vi "Actor Core.vi"(8 "error in":errorcluster, 11 "VG-VNA_GUI in":refnum<class "VG-VNA_GUI.lvclass">) -> (0 "error out":errorcluster, 3 "Actor out":refnum<class "Actor.lvclass">)   [LabVIEW 2020, in "VG-VNA_GUI.lvlib" / "VG-VNA_GUI.lvclass"]
doc: "(<B>Filename</B>: Actor Framework.lvlib:Actor.lvclass:Actor Core.vi)\n\nReceives messages to the actor, reacts to them, and initiates any error handling that may shut the actor down.\n\nDescendant classes may override this VI to append parallel tasks for the actor to complete while it handles messages. Overrides use the Call Parent Class Method node."
uses:
  VG-VNA_GUI.lvclass
  C:/Program Files (x86)/National Instruments/LabVIEW 2020/vi.lib/ActorFramework/Actor/Actor.lvclass
  <vilib>/ActorFramework/Actor/Actor.lvclass
  classes/vna-drivers/liteVNA/VD-connection_settings.ctl
  classes/hardware-protocol/serial/HP-S-baudrate.ctl
  classes/vna-drivers/liteVNA/VD-settingsEasy.ctl
  classes/vna-drivers/liteVNA/VD-sampleSize.ctl
  VG-main_tab.ctl
  VG-sec_tab.ctl
  classes/vna-drivers/liteVNA/VD-settings_status.ctl
  data_handler/VDH-VNA_data_handler/VDH-VNA_data_handler/VDH-calibration_status.ctl
  data_handler/VDH-VNA_data_handler/VDH-VNA_data_handler/VDH-SOLT_calib_Status.ctl
  data_handler/VDH-VNA_data_handler/VDH-VNA_data_handler/VDH-Calibration_prosess.ctl
  data_handler/VDH-VNA_data_handler/VDH-VNA_data_handler/VDH-Calibration_enum.ctl
  hardware_manager/VHM-VNA_Hardware_Manager/VHM-VNA_Hardware_Manager/VHM-connection_status.ctl
  hardware_manager/VHM-VNA_Hardware_Manager/VHM-VNA_Hardware_Manager/VHM-continuous_get_clust.ctl
  VG-file_name_choices.ctl
  VG-data_format_selector.ctl
  VG-VNA_GUI.lvclass/VG-VNA_GUI.ctl
  hardware_manager/VHM-VNA_Hardware_Manager/VHM-VNA_Hardware_Manager Messages/VHM-connectionSettings Msg/VHM-connectionSettings Msg.lvclass/VHM-connectionSettings Msg.ctl
  <vilib>/ActorFramework/Message Enqueuer/Message Enqueuer.lvclass/Message Enqueuer.ctl
  hardware_manager/VHM-VNA_Hardware_Manager/VHM-VNA_Hardware_Manager Messages/VHM-continiousDataSet Msg/VHM-continiousDataSet Msg.lvclass/VHM-continiousDataSet Msg.ctl
  hardware_manager/VHM-VNA_Hardware_Manager/VHM-VNA_Hardware_Manager Messages/VHM-setSettings Msg/VHM-setSettings Msg.lvclass/VHM-setSettings Msg.ctl
  data_handler/VDH-VNA_data_handler/VDH-VNA_data_handler Messages/VDH-loadCalibration Msg/VDH-loadCalibration Msg.lvclass/VDH-loadCalibration Msg.ctl
  data_handler/VDH-VNA_data_handler/VDH-VNA_data_handler/VDH-save_parameters.ctl
  data_handler/VDH-VNA_data_handler/VDH-VNA_data_handler Messages/VDH-RequestSaveData Msg/VDH-RequestSaveData Msg.lvclass/VDH-RequestSaveData Msg.ctl
  data_handler/VDH-VNA_data_handler/VDH-VNA_data_handler Messages/VDH-storeCalibration Msg/VDH-storeCalibration Msg.lvclass/VDH-storeCalibration Msg.ctl
  <vilib>/ActorFramework/Actor/Actor.lvclass/Actor.ctl
  <vilib>/ActorFramework/Message Enqueuer/Enqueue.vi
  <vilib>/ActorFramework/Message Enqueuer/Init from Existing Queue.vi
  hardware_manager/VHM-VNA_Hardware_Manager/VHM-VNA_Hardware_Manager Messages/VHM-connectionSettings Msg/VHM-connectionSettings Msg.lvclass
  C:/Program Files (x86)/National Instruments/LabVIEW 2020/vi.lib/ActorFramework/Message/Message.lvclass
  hardware_manager/VHM-VNA_Hardware_Manager/VHM-VNA_Hardware_Manager Messages/VHM-connect Msg/VHM-connect Msg.lvclass
  hardware_manager/VHM-VNA_Hardware_Manager/VHM-VNA_Hardware_Manager Messages/VHM-getDataSet Msg/VHM-getDataSet Msg.lvclass
  hardware_manager/VHM-VNA_Hardware_Manager/VHM-VNA_Hardware_Manager Messages/VHM-continiousDataSet Msg/VHM-continiousDataSet Msg.lvclass
  hardware_manager/VHM-VNA_Hardware_Manager/VHM-VNA_Hardware_Manager Messages/VHM-disconnect Msg/VHM-disconnect Msg.lvclass
  hardware_manager/VHM-VNA_Hardware_Manager/VHM-VNA_Hardware_Manager Messages/VHM-setSettings Msg/VHM-setSettings Msg.lvclass
  data_handler/VDH-VNA_data_handler/VDH-VNA_data_handler Messages/VDH-generateCalibrationSOLT Msg/VDH-generateCalibrationSOLT Msg.lvclass
  data_handler/VDH-VNA_data_handler/VDH-VNA_data_handler Messages/VDH-loadCalibration Msg/VDH-loadCalibration Msg.lvclass
  data_handler/VDH-VNA_data_handler/VDH-VNA_data_handler Messages/VDH-RequestSaveData Msg/VDH-RequestSaveData Msg.lvclass
  data_handler/VDH-VNA_data_handler/VDH-VNA_data_handler Messages/VDH-RequestStopSaveData Msg/VDH-RequestStopSaveData Msg.lvclass
  data_handler/VDH-VNA_data_handler/VDH-VNA_data_handler Messages/VDH-storeCalibration Msg/VDH-storeCalibration Msg.lvclass
  <vilib>/ActorFramework/Stop Msg/Stop Msg.lvclass
  <vilib>/ActorFramework/Message Priority Queue/Priority Enqueue.vi
  <userlib>/_OpenG.lib/file/file.llb/Valid Path - Traditional__ogtk.vi
  <vilib>/ActorFramework/Message Enqueuer/Message Enqueuer.lvclass
  classes/vna-drivers/liteVNA/VD-LV-LiteVNA.lvclass
  data_handler/VDH-VNA_data_handler/VDH-VNA_data_handler/VDH-VNA_data_handler.lvclass
  hardware_manager/VHM-VNA_Hardware_Manager/VHM-VNA_Hardware_Manager/VHM-VNA_Hardware_Manager.lvclass
  common/features/CF-common_features.lvlib
  <userlib>/_OpenG.lib/file/file.llb/openg_file.lvlib
  classes/hardware-protocol/serial/HP-S-Serial.lvclass
panel:
  in  "Tab Control":enum32{"Main", "Graph"}(tab)
  in  "Main Tab":T1
  in  "autosetup":bool
  in  "connection settings":T2={"Com"="", "baud rate (9600)"=38400} {"baud rate (9600)" items=["75"=75, "110"=110, "134"=134, "150"=150, "300"=300, "600"=600, "1200"=1200, "1800"=1800, "2400"=2400, "4800"=4800, "7200"=7200, "9600"=9600, "14400"=14400, "19200"=19200, "28800"=28800, "38400"=38400, "56000"=56000, "57600"=57600, "115200"=115200, "128000"=128000, "230400"=230400]}
  in  "Connect":bool
  in  "Disconnect":bool
  in  "Set connection settings":bool
  out "connection status":T4
  in  "get set":bool
  in  "Size in sets (0=Until stop)":u8=1
  in  "Stop Reading":bool
  in  "Start Reading":bool
  in  "Stop Saving":bool
  in  "Save Data":bool
  out "Saving Data":bool
  in  "settings":T5={"Start [hz]"=1000000, "Stop [hz]"=5000000, "sampleSize"=101} {"sampleSize" items=["101"=101, "201"=201, "401"=401, "601"=601, "801"=801, "1001"=1001]; "Stop [hz]" format="%.0p"; "Start [hz]" format="%.0p"}
  in  "Set Settings":bool
  in  "Saving name":string="noname"
  in  "Saving path":path
  in  "get cont set":bool
  in  "Read Option":T7
  in  "Second Tab":T8
  in  "calib File Path":path
  in  "Load Calibration file":bool
  out "Calibration Status":T9={"Calib Status"={"Short"=FALSE, "Open"=FALSE, "Load"=FALSE, "Through"=FALSE}, "Calibrated?"=FALSE, "Permativity?"=FALSE, "Progress"={"Progress"=FALSE, "current"=enum."Short", "samples to get"=0}}
  in  "T":bool
  in  "L":bool
  in  "O":bool
  in  "S":bool
  in  "Gen Calib":bool
  in  "Refresh Filename":bool
  out "Filepath":path
  in  "file name choises":T13={"Date"=TRUE, "Time"=TRUE, "Measurement settings"=TRUE, "SOLT?"=TRUE}
  out "File name":string="default_calibration_name"
  in  "Custom filename Part":string
  in  "Save Calibration":bool
  in  "comment":string="Comment"
  in  "Calibration folder Path":path
  out "XY Graph":cluster{u64[], dbl[]}[](graph)
  out "XY Graph 2":cluster{u64[], dbl[]}[](graph)
  out "Settings status":T14
  in  "data format":T15
  in  "Tab Control 2":enum32{"Page 1", "Page 2"}(tab)
  out "XY Graph 3":cluster{u64[], dbl[]}[](graph)
  out "Smith Plot":picture
  out "size(s)":i32
  out "Connected?":bool
  in  "Stop":bool
  out "error IO":errorcluster
  out "current time":timestamp
  # "Manual"
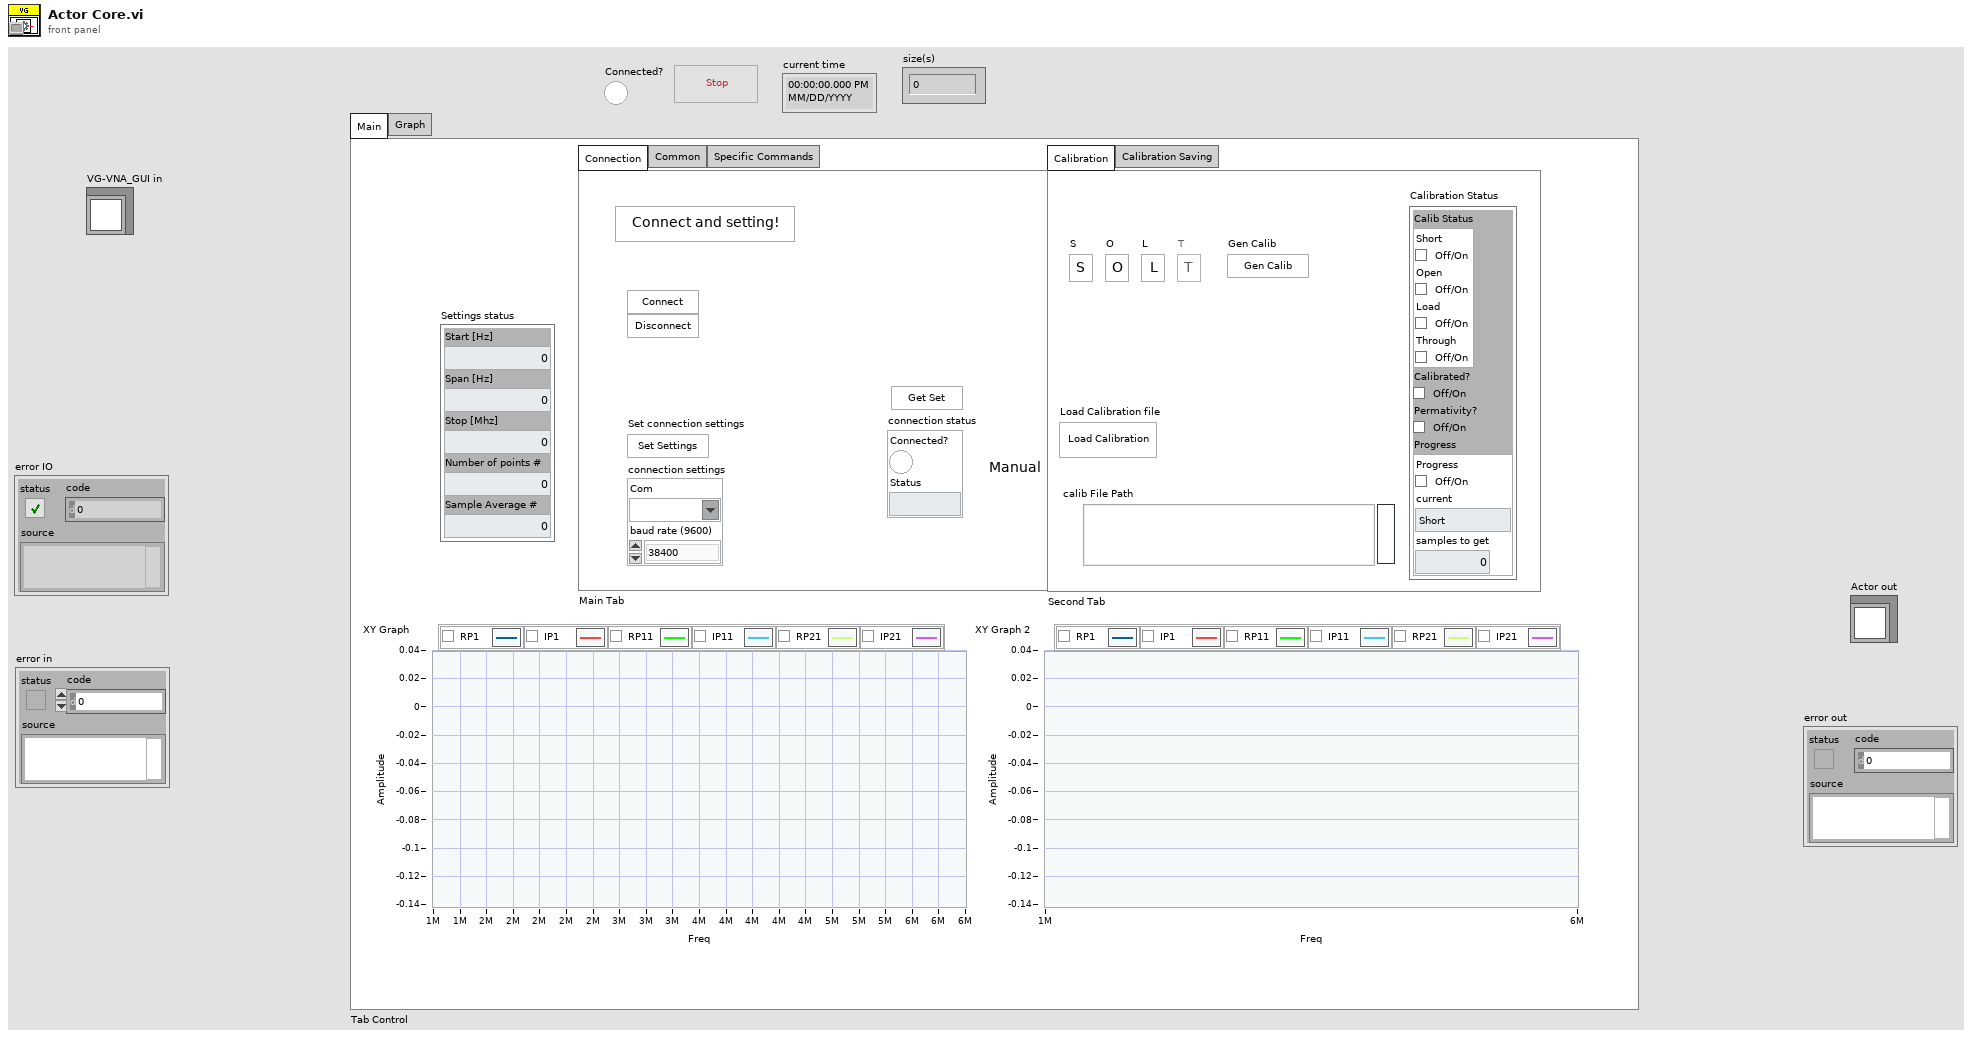
[diagram p1: front panel]
types:
  T1 = typedef "VG-VNA_GUI.lvlib/VG-VNA_GUI.lvclass/VG-main_tab.ctl" = enum32{"Connection", "Common", "Specific Commands"}
  T2 = typedef "VD-LV-LiteVNA.lvclass/VD-connection_settings.ctl" = cluster{"Com":refnum<visa-resource-name>, "baud rate (9600)":T3}
  T3 = typedef "HP-S-Serial.lvclass/HP-S-baudrate.ctl" = u32
  T4 = typedef "VHM-VNA_Hardware_Manager.lvlib/VHM-VNA_Hardware_Manager.lvclass/VHM-connection_status.ctl" = cluster{"Connected?":bool, "Status":string}
  T5 = typedef "VD-LV-LiteVNA.lvclass/VD-settingsEasy.ctl" = cluster{"Start [hz]":u64, "Stop [hz]":u64, "sampleSize":T6}
  T6 = typedef "VD-LV-LiteVNA.lvclass/VD-sampleSize.ctl" = u16
  T7 = typedef "VHM-VNA_Hardware_Manager.lvlib/VHM-VNA_Hardware_Manager.lvclass/VHM-continuous_get_clust.ctl" = cluster{"Amount(0=Continious)":u8, "Start? (false=stop)":bool}
  T8 = typedef "VG-VNA_GUI.lvlib/VG-VNA_GUI.lvclass/VG-sec_tab.ctl" = enum32{"Calibration", "Calibration Saving"}
  T9 = typedef "VDH-VNA_data_handler.lvlib/VDH-VNA_data_handler.lvclass/VDH-calibration_status.ctl" = cluster{"Calib Status":T10, "Calibrated?":bool, "Permativity?":bool, "Progress":T11}
  T10 = typedef "VDH-VNA_data_handler.lvlib/VDH-VNA_data_handler.lvclass/VDH-SOLT_calib_Status.ctl" = cluster{"Short":bool, "Open":bool, "Load":bool, "Through":bool}
  T11 = typedef "VDH-VNA_data_handler.lvlib/VDH-VNA_data_handler.lvclass/VDH-Calibration_prosess.ctl" = cluster{"Progress":bool, "current":T12, "samples to get":u8}
  T12 = typedef "VDH-VNA_data_handler.lvlib/VDH-VNA_data_handler.lvclass/VDH-Calibration_enum.ctl" = enum16{"Non", "Short", "Open", "Load", "Through", "Permativity"}
  T13 = typedef "VG-VNA_GUI.lvlib/VG-VNA_GUI.lvclass/VG-file_name_choices.ctl" = cluster{"Date":bool, "Time":bool, "Measurement settings":bool, "SOLT?":bool}
  T14 = typedef "VD-LV-LiteVNA.lvclass/VD-settings_status.ctl" = cluster{"Start [Hz]":u64, "Span [Hz]":u64, "Stop [Mhz]":u64, "Number of points #":u16, "Sample Average #":u16}
  T15 = typedef "VG-VNA_GUI.lvlib/VG-VNA_GUI.lvclass/VG-data_format_selector.ctl" = cluster{"Complex":bool, "Impedance":bool, "Admittance":bool, "Polar":bool, "Polar Deg":bool, "|Impedance|":bool, "Return Loss":bool}
  T16 = cluster{"Stop":refnum<user-event>, "Graph Data":refnum<user-event>, "Settings status":refnum<user-event>, "Calibration Status":refnum<user-event>, "connection status":refnum<user-event>, "Store Calibration":refnum<user-event>, "Saving Data":refnum<user-event>}
  T17 = typedef "VDH-VNA_data_handler.lvlib/VDH-VNA_data_handler.lvclass/VDH-save_parameters.ctl" = cluster{"Size in sets (0=Until stop)":u8, "Folder Path":path, "filename":string}
  T18 = typedef "VG-VNA_GUI.lvlib/VG-VNA_GUI.lvclass/VG-graph_data.ctl" = cluster{u64[], dbl[]}[]
  T19 = typedef "LVBoundsTypeDef.ctl" = cluster{"Width":u32, "Height":u32}
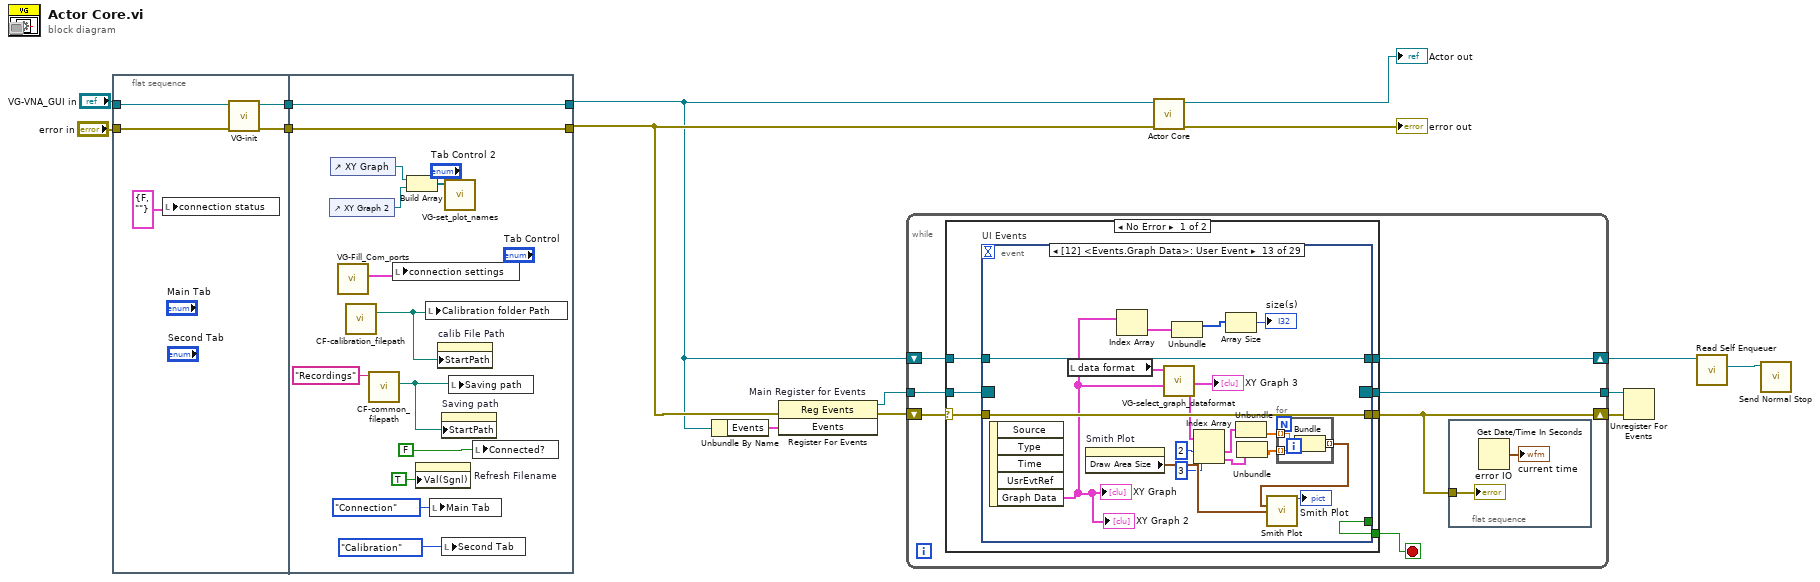
[diagram p0: block diagram]
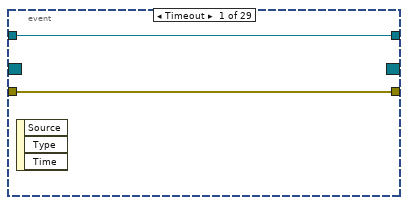
[diagram p2: hidden frame]
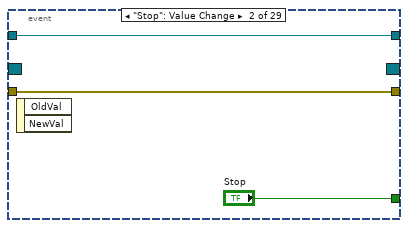
[diagram p3: hidden frame]
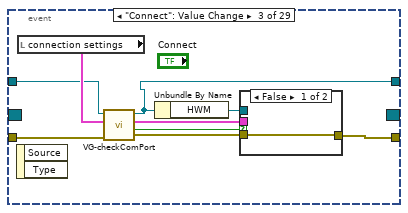
[diagram p4: hidden frame]
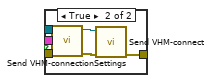
[diagram p5: hidden frame]
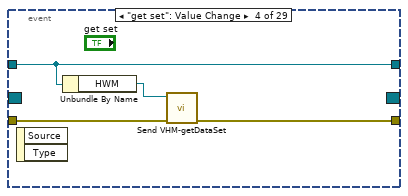
[diagram p6: hidden frame]
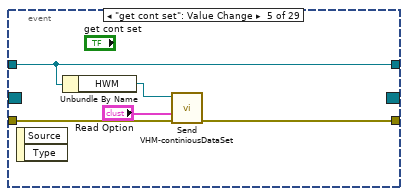
[diagram p7: hidden frame]
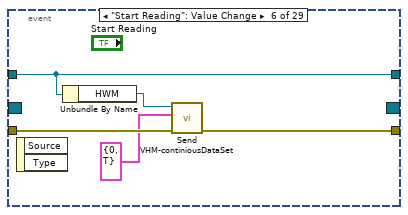
[diagram p8: hidden frame]
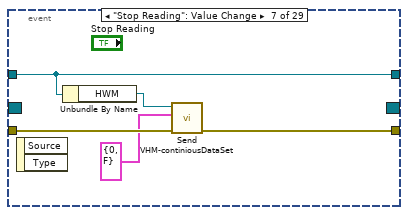
[diagram p9: hidden frame]
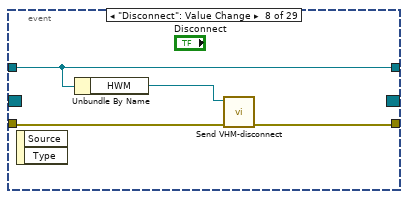
[diagram p10: hidden frame]
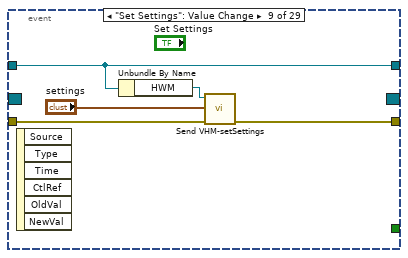
[diagram p11: hidden frame]
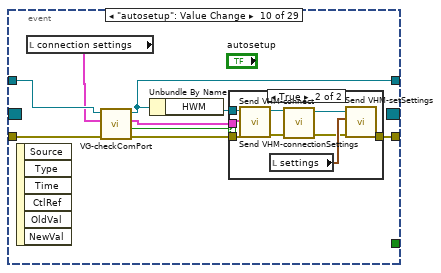
[diagram p12: hidden frame]
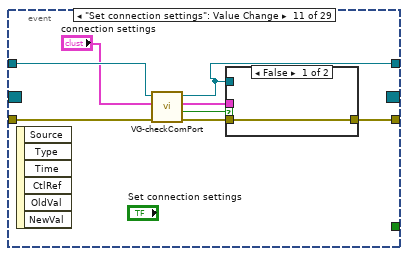
[diagram p14: hidden frame]
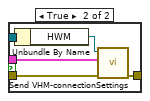
[diagram p15: hidden frame]
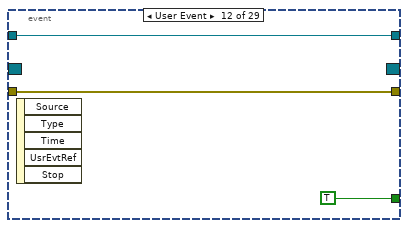
[diagram p16: hidden frame]
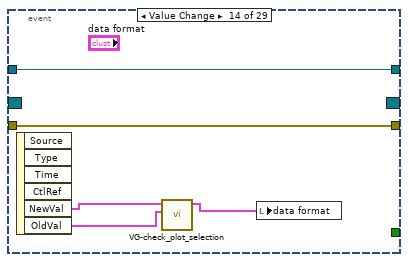
[diagram p17: hidden frame]
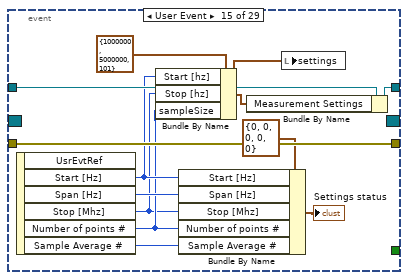
[diagram p18: hidden frame]
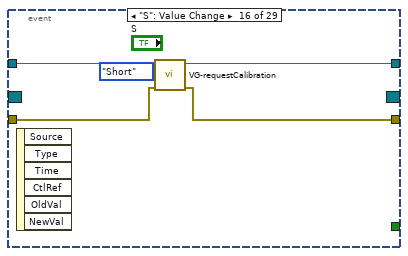
[diagram p19: hidden frame]
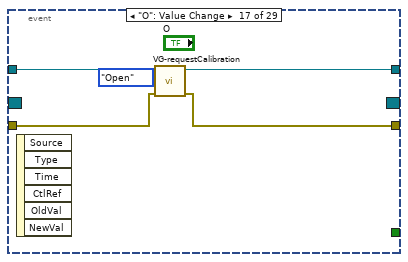
[diagram p20: hidden frame]
diagram:
  n1 = flat-sequence {
    tunnel: "VG-VNA_GUI in" -> [w20]
    tunnel: "error in" -> [w19]
    tunnel: [w18] -> w2
    tunnel: [w17] -> w1
    tunnel: [w32] -> w3
    tunnel: [w33] -> w4
    tunnel: w2 -> [w33]
    tunnel: w1 -> [w32]
    frame #0 {
      n2 = local write "connection status"(T4 {"Connected?"=FALSE, "Status"=""} ("connection status")) -> ()
      n3 = call "VG-init.vi"("error in (no error)"=w19, "VG-VNA_GUI in"=w20) -> ("error out"=w18:errorcluster, "VG-VNA_GUI out"=w17:refnum<class "VG-VNA_GUI.lvclass">)  [unwired: 8 in]
    }
    frame #1 {
      n4 = control-ref of="XY Graph 2"() -> (w30:refnum<vi>)
      n5 = control-ref of="XY Graph"() -> (w29:refnum<vi>)
      n6 = call "VG-Fill_Com_ports.vi"() -> ("output cluster"=w28:T2)  [unwired: 11 in]
      n7 = call "CF-calibration_filepath.vi"() -> ("calibration Path"=w25:path)  [unwired: 10 in, 1 out]
      n8 = call "CF-common_filepath.vi"("Input path"="Recordings") -> ("Common Path + input"=w24:path)  [unwired: 9 in, 1 out]
      n9 = local write "connection settings"(w28) -> ()
      n10 = Build Array(w29, w30) -> (w31:refnum<vi>[])
      n11 = property on="Refresh Filename" class="Bool (strict)"("Val(Sgnl)"=TRUE ("Value (Signaling)")) -> ()  [unwired: 2 in, 2 out]
      n12 = local write "Calibration folder Path"(w25) -> ()
      n13 = local write "Main Tab"(VG-main_tab."Connection" ("Main Tab")) -> ()
      n14 = property on="calib File Path" class="Path"("StartPath"=w25) -> ()  [unwired: 2 in, 2 out]
      n15 = property on="Saving path" class="Path"("StartPath"=w24) -> ()  [unwired: 2 in, 2 out]
      n16 = local write "Second Tab"(VG-sec_tab."Calibration" ("Second Tab")) -> ()
      n17 = call "VG-set_plot_names.vi"("appended array"=w31) -> ()  [unwired: 11 in]
      n18 = local write "Saving path"(w24) -> ()
      n19 = local write "Connected?"(FALSE ("Connected?")) -> ()
    }
  }
  n20 = Unbundle By Name(w3) -> ("Events"=w8:T16)
  n21 = register-events "Main Register for Events"(error in=w4, w8) -> (reference out=w7:refnum<event-registration>, error out=w9:errorcluster)  [unwired: 1 in]
  n22 = while {
    shift-right: [w38] -> w11
    shift-left: w9 -> [w39]
    shift-right: [w36] -> w13
    shift-left: w3 -> [w37]
    tunnel: [w35] -> w10
    tunnel: w7 -> [w34]
    stop <- w40 stop-if-true
    n23 = case shown="No Error" w39 {
      selector: w39 -> [w49 w271]
      tunnel: [w47 TRUE] -> w40
      tunnel: [w48 w271] -> w38
      tunnel: w37 -> [w46 w270]
      tunnel: [w45 w270] -> w36
      tunnel: [w44 w269] -> w35
      tunnel: w34 -> [w43 w269]
      frame No Error {
        n24 = event "UI Events" shown="[12] <Events.Graph Data>: User Event" {
          selector: w43 -> [_ _ _ _ _ _ _ _ _ _ _ _ _ _ _ _ _ _ _ _ _ _ _ _ _ _ _ _ _]
          dyn-events: [_ _ _ _ _ _ _ _ _ _ _ _ _ _ _ _ _ _ _ _ _ _ _ _ _ _ _ _ _] -> w44
          timeout: _ -> [_ _ _ _ _ _ _ _ _ _ _ _ _ _ _ _ _ _ _ _ _ _ _ _ _ _ _ _ _]
          tunnel: w49 -> [w51 w53 w61 w73 w78 w83 w88 w92 w98 w102 w124 w134 w151 w159 w171 w173 w178 w183 w188 w193 w201 w206 w220 w226 w235 w244 w250 w256 w268]
          tunnel: [w51 w53 w63 w71 w76 w81 w86 w90 w97 w106 w125 w134 w151 w159 w171 w174 w179 w184 w189 w192 w198 w205 w219 w225 w235 w244 w250 w253 w268] -> w48
          tunnel: [_ "Stop" _ _ _ _ _ _ _ _ _ TRUE ("Stop") _ _ _ _ _ _ _ _ _ _ _ _ _ _ _ _ _] -> w47
          tunnel: w46 -> [w50 w52 w59 w74 w79 w84 w89 w93 w95 w105 w119 w133 w146 w158 w170 w176 w181 w186 w191 w194 w199 w207 w222 w223 w234 w243 w249 w257 w267]
          tunnel: [w50 w52 w58 w74 w79 w84 w89 w93 w95 w104 w120 w133 w146 w158 w161 w175 w180 w185 w190 w194 w199 w207 w222 w223 w233 w237 w249 w254 w267] -> w45
          event Timeout {
            n25 = event-data() -> ()  [unwired: 1 in, 3 out]
          }
          event "Stop": Value Change {
            n26 = event-data() -> ()  [unwired: 1 in, 2 out]
          }
          event "Connect": Value Change {
            n27 = event-data() -> ()  [unwired: 1 in, 2 out]
            n28 = local read "connection settings"() -> (w60:T2)
            n29 = call "VG-checkComPort.vi"("error in (no error)"=w61, "connection settings"=w60, "VG-VNA_GUI in"=w59) -> ("error out"=w56:errorcluster, "Com Port Found?"=w55:bool, "connection settings dup"=w57:T2, "VG-VNA_GUI out"=w58:refnum<class "VG-VNA_GUI.lvclass">)  [unwired: 5 in]
            n30 = Unbundle By Name(w58) -> ("HWM"=w62:refnum<class "Message Enqueuer.lvclass">)
            n31 = case shown="False" w55 {
              tunnel: [w64 w70] -> w63
              tunnel: w62 -> [_ w69]
              tunnel: w57 -> [_ w67]
              tunnel: w56 -> [w64 w66]
              frame False {
              }
              frame True {
                n32 = call "Send VHM-connectionSettings.vi"("error in (no error)"=w66, "connection settings"=w67, "Message Enqueuer"=w69) -> ("error out"=w65:errorcluster, "Message Enqueuer out"=w68:refnum<class "Message Enqueuer.lvclass">)  [unwired: 7 in]
                n33 = call "Send VHM-connect.vi"("error in (no error)"=w65, "Message Enqueuer"=w68) -> ("error out"=w70:errorcluster)  [unwired: 8 in, 1 out]
              }
            }
          }
          event "get set": Value Change {
            n34 = event-data() -> ()  [unwired: 1 in, 2 out]
            n35 = Unbundle By Name(w74) -> ("HWM"=w72:refnum<class "Message Enqueuer.lvclass">)
            n36 = call "Send VHM-getDataSet.vi"("error in (no error)"=w73, "Message Enqueuer"=w72) -> ("error out"=w71:errorcluster)  [unwired: 8 in, 1 out]
          }
          event "get cont set": Value Change {
            n37 = event-data() -> ()  [unwired: 1 in, 2 out]
            n38 = Unbundle By Name(w79) -> ("HWM"=w77:refnum<class "Message Enqueuer.lvclass">)
            n39 = call "Send VHM-continiousDataSet.vi"("error in (no error)"=w78, "Read Option"="Read Option", "Message Enqueuer"=w77) -> ("error out"=w76:errorcluster)  [unwired: 7 in, 1 out]
          }
          event "Start Reading": Value Change {
            n40 = event-data() -> ()  [unwired: 1 in, 2 out]
            n41 = Unbundle By Name(w84) -> ("HWM"=w82:refnum<class "Message Enqueuer.lvclass">)
            n42 = call "Send VHM-continiousDataSet.vi"("error in (no error)"=w83, "Read Option"=T7 {"Amount(0=Continious)"=0, "Start? (false=stop)"=TRUE} ("Read Option 2"), "Message Enqueuer"=w82) -> ("error out"=w81:errorcluster)  [unwired: 7 in, 1 out]
          }
          event "Stop Reading": Value Change {
            n43 = event-data() -> ()  [unwired: 1 in, 2 out]
            n44 = Unbundle By Name(w89) -> ("HWM"=w87:refnum<class "Message Enqueuer.lvclass">)
            n45 = call "Send VHM-continiousDataSet.vi"("error in (no error)"=w88, "Read Option"=T7 {"Amount(0=Continious)"=0, "Start? (false=stop)"=FALSE} ("Read Option 2"), "Message Enqueuer"=w87) -> ("error out"=w86:errorcluster)  [unwired: 7 in, 1 out]
          }
          event "Disconnect": Value Change {
            n46 = event-data() -> ()  [unwired: 1 in, 2 out]
            n47 = Unbundle By Name(w93) -> ("HWM"=w91:refnum<class "Message Enqueuer.lvclass">)
            n48 = call "Send VHM-disconnect.vi"("error in (no error)"=w92, "Message Enqueuer"=w91) -> ("error out"=w90:errorcluster)  [unwired: 8 in, 1 out]
          }
          event "Set Settings": Value Change {
            n49 = event-data() -> ()  [unwired: 1 in, 6 out]
            n50 = Unbundle By Name(w95) -> ("HWM"=w94:refnum<class "Message Enqueuer.lvclass">)
            n51 = call "Send VHM-setSettings.vi"("error in (no error)"=w98, "settings"="settings", "Message Enqueuer"=w94) -> ("error out"=w97:errorcluster)  [unwired: 7 in, 1 out]
          }
          event "autosetup": Value Change {
            n52 = event-data() -> ()  [unwired: 1 in, 6 out]
            n53 = local read "connection settings"() -> (w99:T2)
            n54 = call "VG-checkComPort.vi"("error in (no error)"=w102, "connection settings"=w99, "VG-VNA_GUI in"=w105) -> ("error out"=w103:errorcluster, "Com Port Found?"=w100:bool, "connection settings dup"=w101:T2, "VG-VNA_GUI out"=w104:refnum<class "VG-VNA_GUI.lvclass">)  [unwired: 5 in]
            n55 = Unbundle By Name(w104) -> ("HWM"=w107:refnum<class "Message Enqueuer.lvclass">)
            n56 = case shown="True" w100 {
              tunnel: w107 -> [_ w116]
              tunnel: [w108 w111] -> w106
              tunnel: w103 -> [w108 w110]
              tunnel: w101 -> [_ w109]
              frame False {
              }
              frame True {
                n57 = call "Send VHM-connectionSettings.vi"("error in (no error)"=w110, "connection settings"=w109, "Message Enqueuer"=w116) -> ("error out"=w115:errorcluster, "Message Enqueuer out"=w114:refnum<class "Message Enqueuer.lvclass">)  [unwired: 7 in]
                n58 = local read "settings"() -> (w117:T5)
                n59 = call "Send VHM-connect.vi"("error in (no error)"=w115, "Message Enqueuer"=w114) -> ("error out"=w112:errorcluster, "Message Enqueuer out"=w113:refnum<class "Message Enqueuer.lvclass">)  [unwired: 8 in]
                n60 = call "Send VHM-setSettings.vi"("error in (no error)"=w112, "settings"=w117, "Message Enqueuer"=w113) -> ("error out"=w111:errorcluster)  [unwired: 7 in, 1 out]
              }
            }
          }
          event "Set connection settings": Value Change {
            n61 = event-data() -> ()  [unwired: 1 in, 6 out]
            n62 = call "VG-checkComPort.vi"("error in (no error)"=w124, "connection settings"="connection settings", "VG-VNA_GUI in"=w119) -> ("error out"=w123:errorcluster, "Com Port Found?"=w121:bool, "connection settings dup"=w122:T2, "VG-VNA_GUI out"=w120:refnum<class "VG-VNA_GUI.lvclass">)  [unwired: 5 in]
            n63 = case shown="False" w121 {
              tunnel: w120 -> [_ w131]
              tunnel: w122 -> [_ w129]
              tunnel: w123 -> [w126 w128]
              tunnel: [w126 w127] -> w125
              frame False {
              }
              frame True {
                n64 = Unbundle By Name(w131) -> ("HWM"=w130:refnum<class "Message Enqueuer.lvclass">)
                n65 = call "Send VHM-connectionSettings.vi"("error in (no error)"=w128, "connection settings"=w129, "Message Enqueuer"=w130) -> ("error out"=w127:errorcluster)  [unwired: 7 in, 1 out]
              }
            }
          }
          event User Event {
            n66 = event-data() -> ()  [unwired: 1 in, 5 out]
          }
          event User Event {
            n67 = event-data() -> ("Graph Data"=w147:T18)  [unwired: 1 in, 4 out]
            "XY Graph" <- w147
            "XY Graph 2" <- w147
            n68 = local read "data format"() -> (w145:T15)
            n69 = property on="Smith Plot" class="Pict"() -> ("Draw Area Size"=w143:T19)  [unwired: 2 in, 2 out]
            n70 = Index Array(array=w147) -> (element=w150:cluster{u64[], dbl[]})  [unwired: 1 in]
            n71 = call "VG-select_graph_dataformat.vi"("Graph Data"=w147, "data format"=w145) -> ("Graph Data out"=w142:T18)  [unwired: 9 in]
            "XY Graph 3" <- w142
            n72 = Unbundle(w150) -> (w149:u64[])  [unwired: 1 out]
            n73 = Index Array(array=w142, index #1=2 ("index"), index #2=3 ("index")) -> (element #1=w139:cluster{u64[], dbl[]}, element #2=w138:cluster{u64[], dbl[]})
            n74 = Array Size(array=w149) -> (size(s)=→"size(s)":i32)
            n75 = Unbundle(w139) -> (w137:dbl[])  [unwired: 1 out]
            n76 = Unbundle(w138) -> (w136:dbl[])  [unwired: 1 out]
            n77 = for {
              tunnel: w137 -> [w154] mode=indexing
              tunnel: w136 -> [w153] mode=indexing
              tunnel: [w152] -> w135 mode=indexing
              n78 = Bundle(w154, w153) -> (w152:cluster{dbl, dbl})  [unwired: 1 in]
            }
            n79 = call <vilib>:"Smith Plot.vi"("smith plot"=w135, "dimensions (w,h)"=w143) -> ("new picture"=→"Smith Plot":picture)  [unwired: 13 in]
          }
          event Value Change {
            n80 = event-data() -> ("NewVal"=w157:T15, "OldVal"=w156:T15)  [unwired: 1 in, 4 out]
            n81 = call "VG-check_plot_selection.vi"("data format Last"=w156, "data format"=w157) -> ("data format out"=w155:T15)  [unwired: 9 in]
            n82 = local write "data format"(w155) -> ()
          }
          event User Event {
            n83 = event-data() -> ("Start [Hz]"=w165:u64, "Span [Hz]"=w164:u64, "Stop [Mhz]"=w162:u64, "Number of points #"=w163:u16, "Sample Average #"=w167:u16)  [unwired: 1 in, 1 out]
            n84 = Bundle By Name(cluster=T5 {"Start [hz]"=1000000, "Stop [hz]"=5000000, "sampleSize"=101} ("settings"), "Start [hz]"=w165, "Stop [hz]"=w162, "sampleSize"=w163) -> (w160:T5)
            n85 = Bundle By Name(cluster=T14 {"Start [Hz]"=0, "Span [Hz]"=0, "Stop [Mhz]"=0, "Number of points #"=0, "Sample Average #"=0} ("Settings status"), "Start [Hz]"=w165, "Span [Hz]"=w164, "Stop [Mhz]"=w162, "Number of points #"=w163, "Sample Average #"=w167) -> (→"Settings status":T14)
            n86 = Bundle By Name(cluster=w170, "Measurement Settings"=w160) -> (w161:refnum<class "VG-VNA_GUI.lvclass">)
            n87 = local write "settings"(w160) -> ()
          }
          event "S": Value Change {
            n88 = event-data() -> ()  [unwired: 1 in, 6 out]
            n89 = call "VG-requestCalibration.vi"("error in (no error)"=w173, "Calibration Type"=VDH-Calibration_enum."Short", "VG-VNA_GUI in"=w176) -> ("error out"=w174:errorcluster, "VG-VNA_GUI out"=w175:refnum<class "VG-VNA_GUI.lvclass">)  [unwired: 7 in]
          }
          event "O": Value Change {
            n90 = event-data() -> ()  [unwired: 1 in, 6 out]
            n91 = call "VG-requestCalibration.vi"("error in (no error)"=w178, "Calibration Type"=VDH-Calibration_enum."Open", "VG-VNA_GUI in"=w181) -> ("error out"=w179:errorcluster, "VG-VNA_GUI out"=w180:refnum<class "VG-VNA_GUI.lvclass">)  [unwired: 7 in]
          }
          event "L": Value Change {
            n92 = event-data() -> ()  [unwired: 1 in, 6 out]
            n93 = call "VG-requestCalibration.vi"("error in (no error)"=w183, "Calibration Type"=VDH-Calibration_enum."Load", "VG-VNA_GUI in"=w186) -> ("error out"=w184:errorcluster, "VG-VNA_GUI out"=w185:refnum<class "VG-VNA_GUI.lvclass">)  [unwired: 7 in]
          }
          event "T": Value Change {
            n94 = event-data() -> ()  [unwired: 1 in, 6 out]
            n95 = call "VG-requestCalibration.vi"("error in (no error)"=w188, "Calibration Type"=VDH-Calibration_enum."Through", "VG-VNA_GUI in"=w191) -> ("error out"=w189:errorcluster, "VG-VNA_GUI out"=w190:refnum<class "VG-VNA_GUI.lvclass">)  [unwired: 7 in]
          }
          event "Gen Calib": Value Change {
            n96 = event-data() -> ()  [unwired: 1 in, 6 out]
            n97 = Unbundle By Name(w194) -> ("DH"=w195:refnum<class "Message Enqueuer.lvclass">)
            n98 = call "Send VDH-generateCalibrationSOLT.vi"("error in (no error)"=w193, "Message Enqueuer"=w195) -> ("error out"=w192:errorcluster)  [unwired: 8 in, 1 out]
          }
          event "Save Calibration": Value Change {
            n99 = event-data() -> ()  [unwired: 1 in, 6 out]
            n100 = Unbundle By Name(w199) -> ("Store Calibration"=w197:refnum<user-event>)
            n101 = property on="Refresh Filename" class="Bool (strict)"(error in=w201, "Val(Sgnl)"=TRUE ("Value (Signaling)")) -> (error out=w200:errorcluster)  [unwired: 1 in, 1 out]
            n102 = Generate User Event(user event=w197, event data cluster=FALSE ("event data"), error in=w200) -> (error out=w198:errorcluster)  [unwired: 1 in, 1 out]
          }
          event "Load Calibration file": Value Change {
            n103 = event-data() -> ()  [unwired: 1 in, 6 out]
            n104 = call-poly <userlib>:"Valid Path__ogtk.vi"("path"="calib File Path") -> ("valid"=w203:bool)
            n105 = case shown="False" w203 {
              tunnel: w207 -> [_ w213]
              tunnel: w206 -> [w208 w212]
              tunnel: "calib File Path" -> [_ w211]
              tunnel: [w208 w210] -> w205
              frame False {
              }
              frame True {
                n106 = Unbundle By Name(w213) -> ("DH"=w209:refnum<class "Message Enqueuer.lvclass">)
                n107 = call "Send VDH-loadCalibration.vi"("error in (no error)"=w212, "File path"=w211, "Message Enqueuer"=w209) -> ("error out"=w210:errorcluster)  [unwired: 7 in, 1 out]
              }
            }
          }
          event "Save Data": Value Change {
            n108 = event-data() -> ()  [unwired: 1 in, 6 out]
            n109 = Unbundle By Name(w222) -> ("DH"=w221:refnum<class "Message Enqueuer.lvclass">)
            n110 = Bundle By Name(cluster=T17 {"Size in sets (0=Until stop)"=1, "Folder Path"=path "", "filename"=""} ("Save Parameters"), "Size in sets (0=Until stop)"="Size in sets (0=Until stop)", "Folder Path"="Saving path", "filename"="Saving name") -> (w217:T17)
            n111 = call "Send VDH-RequestSaveData.vi"("error in (no error)"=w220, "Save Parameters"=w217, "Message Enqueuer"=w221) -> ("error out"=w219:errorcluster)  [unwired: 7 in, 1 out]
          }
          event "Stop Saving": Value Change {
            n112 = event-data() -> ()  [unwired: 1 in, 6 out]
            n113 = Unbundle By Name(w223) -> ("DH"=w224:refnum<class "Message Enqueuer.lvclass">)
            n114 = call "Send VDH-RequestStopSaveData.vi"("error in (no error)"=w226, "Message Enqueuer"=w224) -> ("error out"=w225:errorcluster)  [unwired: 8 in, 1 out]
          }
          event "Custom filename Part", "Calibration folder Path", "Refresh Filename": Value Change {
            n115 = event-data() -> ()  [unwired: 1 in, 6 out]
            n116 = call "VG-generateFilePath.vi"("file name choises"="file name choises", "Filename"="Custom filename Part", "Calibration Folder Path"="Calibration folder Path", "VG-VNA_GUI in"=w234) -> ("filename out"=→"File name":string, "filepath"=→"Filepath":path, "VG-VNA_GUI out"=w233:refnum<class "VG-VNA_GUI.lvclass">)  [unwired: 5 in]
            n117 = local write "Refresh Filename"(FALSE ("Refresh Filename")) -> ()
          }
          event User Event {
            n118 = event-data() -> ("Calib Status"=w241:T10, "Calibrated?"=w238:bool, "Permativity?"=w239:bool, "Progress"=w240:T11)  [unwired: 1 in]
            n119 = Bundle By Name(cluster=T9 {"Calib Status"={"Short"=FALSE, "Open"=FALSE, "Load"=FALSE, "Through"=FALSE}, "Calibrated?"=FALSE, "Permativity?"=FALSE, "Progress"={"Progress"=FALSE, "current"=enum."Short", "samples to get"=0}} ("Calibration Status"), "Calib Status"=w241, "Calibrated?"=w238, "Permativity?"=w239, "Progress"=w240) -> (w236:T9)
            "Calibration Status" <- w236
            n120 = Bundle By Name(cluster=w243, "Calibration Status"=w236) -> (w237:refnum<class "VG-VNA_GUI.lvclass">)
          }
          event User Event {
            n121 = event-data() -> ("Connected?"=w245:bool, "Status"=w246:string)  [unwired: 1 in]
            "Connected?" <- w245
            n122 = case shown="True" w245 {
              frame False {
              }
              frame True {
                n123 = First Call?() -> (First Call?: T/F=w251:bool)
                n124 = case shown="True" w251 {
                  frame False {
                  }
                  frame True {
                    n125 = local write "Main Tab"(VG-main_tab."Common" ("Main Tab")) -> ()
                  }
                }
              }
            }
            n126 = Bundle By Name(cluster=T4 {"Connected?"=FALSE, "Status"=""} ("connection status"), "Connected?"=w245, "Status"=w246) -> (→"connection status":T4)
          }
          event User Event {
            n127 = event-data() -> ()  [unwired: 1 in, 1 out]
            n128 = call "VG-verifyCalibrationPath.vi"("error in (no error)"=w256, "VG-VNA_GUI in"=w257) -> ("error out"=w255:errorcluster, "Valid?"=w258:bool, "VG-VNA_GUI out"=w254:refnum<class "VG-VNA_GUI.lvclass">)  [unwired: 7 in]
            n129 = case shown="True" w258 {
              tunnel: w254 -> [_ w265]
              tunnel: w255 -> [w259 w264]
              tunnel: [w259 w262] -> w253
              frame False {
              }
              frame True {
                n130 = Unbundle By Name(w265) -> ("DH"=w263:refnum<class "Message Enqueuer.lvclass">, "Filepath"=w261:path)
                n131 = call "Send VDH-storeCalibration.vi"("error in (no error)"=w264, "comment"="comment", "Calibration File Path"=w261, "Message Enqueuer"=w263) -> ("error out"=w262:errorcluster)  [unwired: 6 in, 1 out]
              }
            }
          }
          event User Event {
            n132 = event-data() -> ("Saving Data"=→"Saving Data":bool)  [unwired: 1 in]
          }
        }
      }
      frame Error {
      }
    }
    n133 = flat-sequence {
      tunnel: w38 -> [w42]
      frame #0 {
        n134 = Get Date/Time In Seconds() -> (seconds since 1Jan1904=→"current time":timestamp)
        "error IO" <- w42
      }
    }
  }
  n135 = call-parent "Actor Core.vi"("error in"=w4, "Actor in"=w3) -> ("error out"=→"error out":errorcluster, "Actor out"=→"Actor out":refnum<class "Actor.lvclass">)  [unwired: 8 in]
  n136 = Unregister For Events(event registration refnum=w10, error in=w11) -> ()  [unwired: 1 out]
  n137 = call <vilib>:"Read Self Enqueuer.vi"("Actor"=w13) -> ("Self Enqueuer"=w12:refnum<class "Message Enqueuer.lvclass">)  [unwired: 10 in]
  n138 = call <vilib>:"Send Normal Stop.vi"("Message Enqueuer"=w12) -> ()  [unwired: 10 in, 1 out]
